vi "FindRowIndex.vi"(8 "error in (no error)":errorcluster, 9 "PartNumberData":T1(array[cluster])=[{"ID"="{A382EAD5-775E-4515-9346-9721282186AB}", "PartNumberRegex"="^J(\\d{11,13}):K(\\d{11,13})$", "Model"="0B", "Suffix"="A1"}, {"ID"="{54D08A76-3C8C-49C7-9978-941D39CDBD69}", "PartNumberRegex"="^(S:\\w{3}\\d{2}\\d{2}(\\d{4}|[[:xdigit:]]{4}))(P:(\\d{8})(\\w{1,2})(\\d{6})(\\d{3}))$", "Model"="0C", "Suffix"="A2"}, {"ID"="{FA4F72A4-5E99-4093-956D-40A0BA740E36}", "PartNumberRegex"="^(P:)(10-000001)(R:)(04)(S:)(QMC220[0-9]+)", "Model"="SubM", "Suffix"="A3"}], 10 "Barcode":string="P:10-000001R:04S:QMC2200185") -> (0 "error out":errorcluster, 1 "SerialNumber":string="QMC2200185", 2 "PartNumber":string="10-000001", 3 "ArrayIndex":i32=2, 5 "Revision":string="04")   [LabVIEW 2021, in "PreUUT.lvclass"]
uses:
  PreUUT.lvclass
  <vilib>/regexp/Match Regular Expression.xnode
panel:
  out "PN_SN":string="P:10-000001R:04S:QMC2200185"
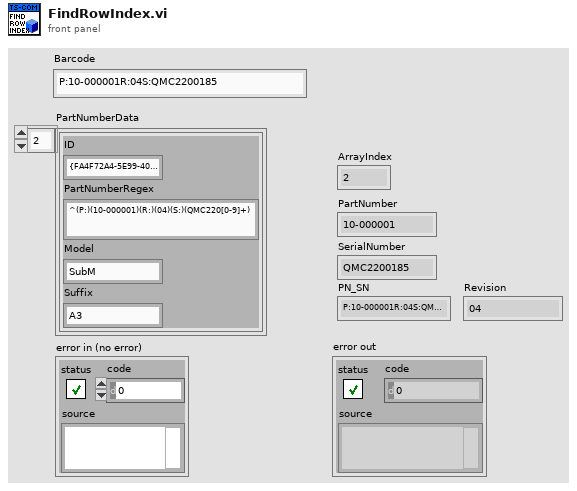
[diagram p1: front panel]
types:
  T1 = cluster{"ID":string, "PartNumberRegex":string, "Model":string, "Suffix":string}[]
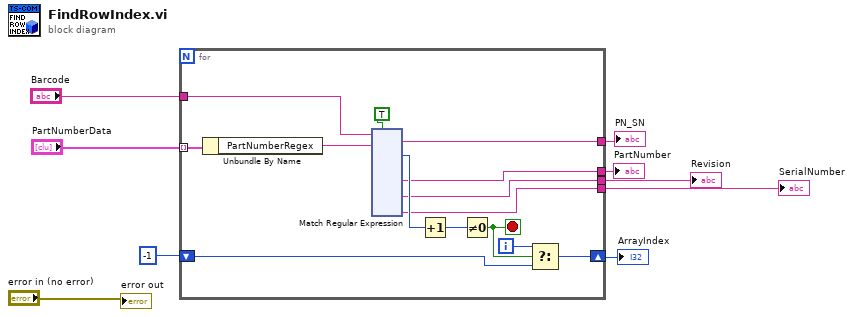
[diagram p0: block diagram]
diagram:
  n1 = for {
    tunnel: "Barcode" -> [w20]
    shift-right: [w16] -> w7
    shift-left: -1 -> [w17]
    tunnel: "PartNumberData" -> [w15] mode=indexing
    tunnel: [w12] -> w5
    tunnel: [w10] -> w4
    tunnel: [w13] -> w3
    tunnel: [w11] -> w2
    i -> [w18]
    stop <- w19 stop-if-true
    n2 = Unbundle By Name(w15) -> ("PartNumberRegex"=w14:string)
    n3 = xnode "Match Regular Expression"("input string"=w20, "regular expression"=w14, "ignore case? (F)"=TRUE) -> ("whole match"=w13:string, "offset past match"=w23:i32, "submatch 2"=w12:string, "submatch 4"=w11:string, "submatch 6"=w10:string)  [unwired: 3 in, 6 out]
    n4 = Increment(x=w23) -> (x+1=w22:i32)
    n5 = Not Equal To 0?(x=w22) -> (x != 0?=w19:bool)
    n6 = Select(t=w18, s=w19, f=w17) -> (s? t:f=w16:i32)
  }
  "ArrayIndex" <- w7
  "PartNumber" <- w5
  "SerialNumber" <- w4
  "PN_SN" <- w3
  "Revision" <- w2
  "error out" <- "error in (no error)"
